vi "OSR_Nu.vi"(2 "Enable?":bool=TRUE, 4 "input":bool) -> (0 "Falling":bool, 1 "Rising":bool)   [LabVIEW 2020]
panel:
  out "error out":errorcluster
  in  "error in (no error)":errorcluster
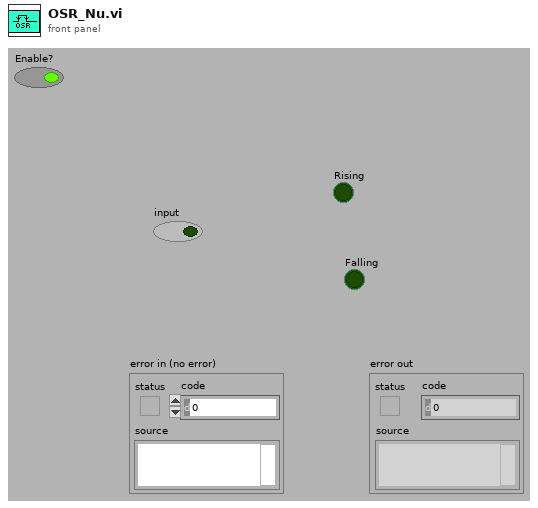
[diagram p1: front panel]
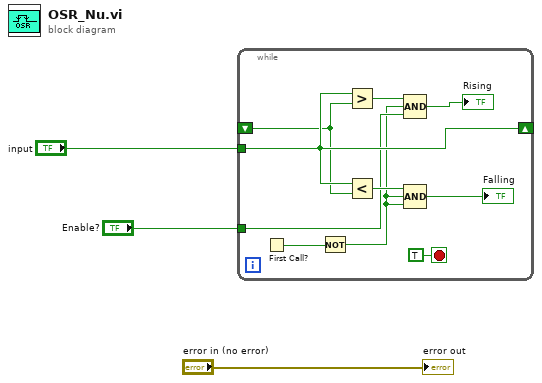
[diagram p0: block diagram]
diagram:
  n1 = while {
    shift-right: [w12] -> _
    shift-left: _ -> [w11]
    tunnel: "input" -> [w12]
    tunnel: "Enable?" -> [w5]
    stop <- TRUE stop-if-true
    n2 = First Call?() -> (First Call?: T/F=w10:bool)
    n3 = Not(x=w10) -> (.not. x?=w4:bool)
    n4 = Greater?(x=w12, y=w11) -> (0:w9:bool)
    n5 = Less?(x=w12, y=w11) -> (x < y?=w7:bool)
    n6 = Compound Arithmetic op=AND(w9, w4, w5) -> (→"Rising":bool)
    n7 = Compound Arithmetic op=AND(w7, w4, w4) -> (→"Falling":bool)
  }
  "error out" <- "error in (no error)"
